vi "Receive Message.vi"(8 "error in (no error)":errorcluster, 9 "timeout in ms (-1)":i32=-1, 11 "Process In":refnum<class "Process.lvclass">) -> (0 "error out":errorcluster, 1 "Message Data":variant, 2 "Message":string, 3 "Process Out":refnum<class "Process.lvclass">)   [LabVIEW 2020, in "Process.lvclass"]
doc: "This VI pulls messages off the Message Queue."
uses:
  Process.lvclass
  Process.lvclass/Process.ctl
  <vilib>/Utility/error.llb/Error Cluster From Error Code.vi
  <vilib>/ErrorRing/Error Ring.xnode
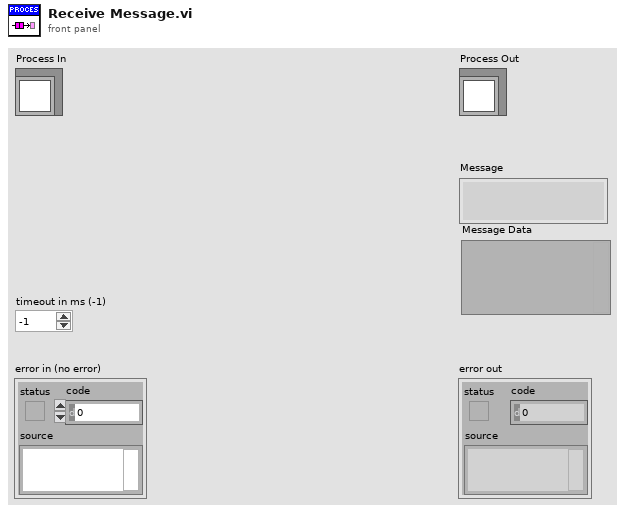
[diagram p1: front panel]
types:
  T1 = typedef "Process.lvclass/Message Cluster.ctl" = cluster{"Message":string, "Message Data":variant, "Request Callback":refnum<class "Callback.lvclass">}
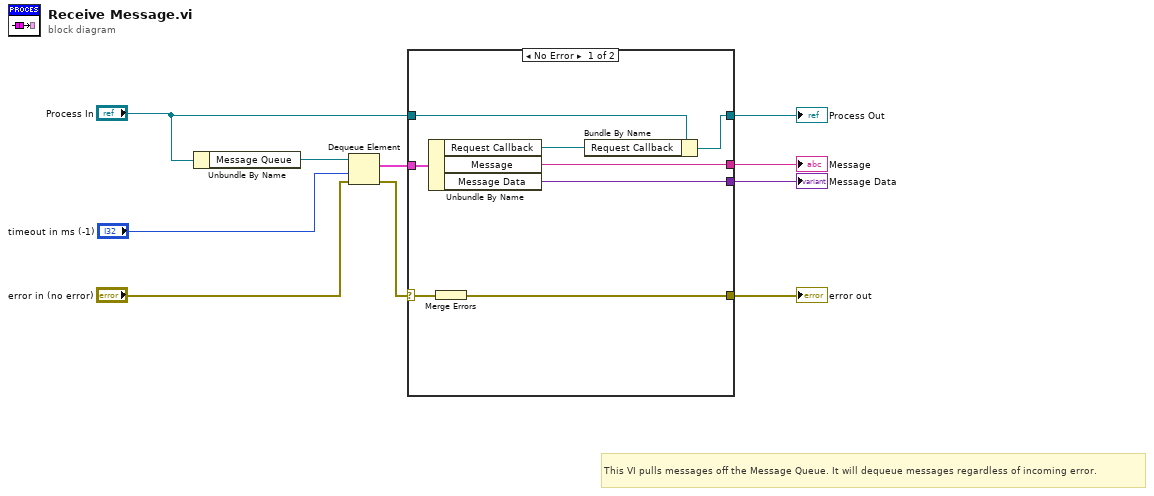
[diagram p0: block diagram]
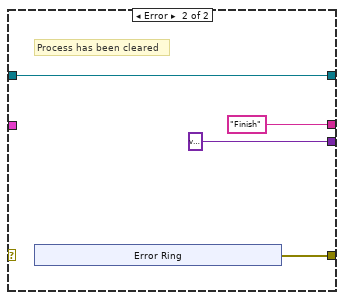
[diagram p2: hidden frame]
diagram:
  # "This VI pulls messages off the Message Queue. It will dequeue messages regardless of incoming error."
  n1 = Unbundle By Name("Process In") -> ("Message Queue"=w10:refnum<queue>)
  n2 = Dequeue Element(queue=w10, timeout in ms (-1)="timeout in ms (-1)", error in (no error)="error in (no error)") -> (element=w4:T1, error out=w5:errorcluster)  [unwired: 2 out]
  n3 = case shown="No Error" w5 {
    selector: w5 -> [w18 _]
    tunnel: [w13 w20] -> w9
    tunnel: [w16 "Finish" ("Message")] -> w8
    tunnel: [w15 variant ("Message Data")] -> w7
    tunnel: w4 -> [w17 _]
    tunnel: [w12 w19] -> w1
    tunnel: "Process In" -> [w14 w19]
    frame No Error {
      n4 = Unbundle By Name(w17) -> ("Request Callback"=w11:refnum<class "Callback.lvclass">, "Message"=w16:string, "Message Data"=w15:variant)
      n5 = Merge Errors(w18) -> (w13:errorcluster)
      n6 = Bundle By Name(cluster=w14, "Request Callback"=w11) -> (w12:refnum<class "Process.lvclass">)
    }
    frame Error {
      # "Process has been cleared"
      n7 = xnode "Error Ring"() -> ("error out"=w20:errorcluster)
    }
  }
  "error out" <- w9
  "Process Out" <- w1
  "Message" <- w8
  "Message Data" <- w7
